vi "Sub Routing program.vi"(0 "queue Out in":refnum<queue>, 1 "FeedBack Channel":string[](array[string]), 2 "Load":refnum<vi>, 5 "reference in":refnum<vi>, 9 "Feature Step Enable":T1(array[cluster]), 11 "error in (no error)":errorcluster, 12 "Str Refnum":refnum<vi>, 13 "Lvdt":refnum<vi>, 14 "Pict Refnum":refnum<vi>) -> (3 "2D Picture":picture, 4 "Queue out":refnum<queue>, 6 "reference out":refnum<vi>, 10 "Result":bool, 15 "error out":errorcluster)   [LabVIEW 2020]
uses:
  Test  enqueue/AutoTest seq.ctl
  Galobal variable_TI.vi
  Project Setup/Globle Variable/GR_Servo.vi
panel:
  out "error out 2":errorcluster
  in  "Select Part":u16(ring) items=["CHECK BARCODE.jpg", "Difusser.jpg", "FIX BLACK PART.jpg", "FIXED PCB.jpg", "INSER KEYPAD.jpg", "IONIZE PCB.jpg", "light box ionization.jpg", "MOVE DOWN PART.jpg", "MOVING PART.jpg", "PART.jpg", "PUT PART ON FIXTURE.jpg"]
  out "Error Message":string
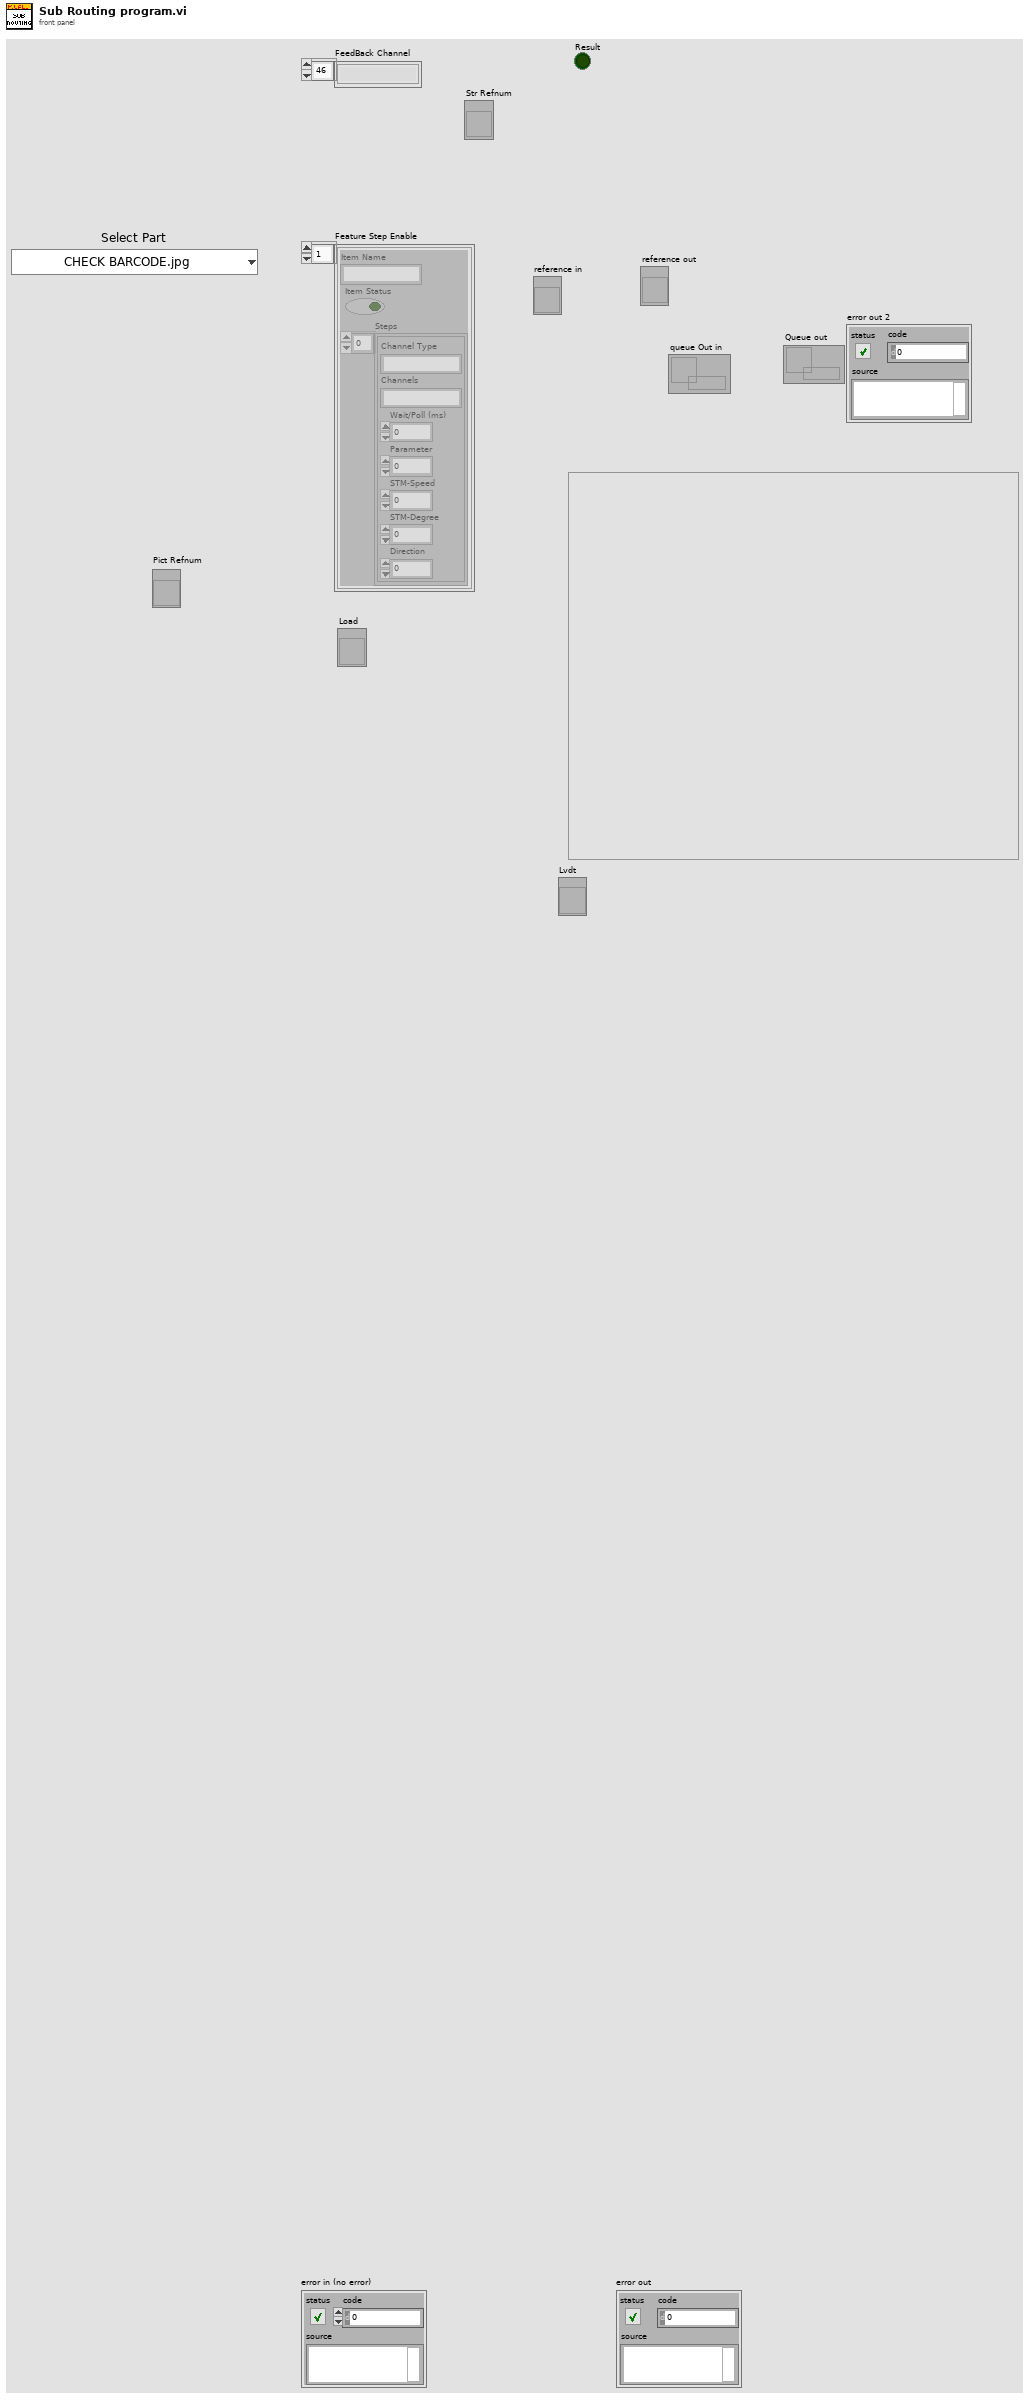
[diagram p1: front panel]
types:
  T1 = cluster{"Item Name":string, "Item Status":bool, "Steps":cluster{"Channel Type":string, "Channels":string, "Wait/Poll (ms)":u32, "Parameter":u8, "STM-Speed":i32, "STM-Degree":u32, "Direction":u8}[]}[]
  T2 = cluster{"Channel Type":string, "Channels":string, "Wait/Poll (ms)":u32, "Parameter":u8, "STM-Speed":i32, "STM-Degree":u32, "Direction":u8}[]
  T3 = cluster{"Start":bool, "Emergency ":bool, "Reset":bool, "Home":bool, "Safety":bool}
  T4 = typedef "LVPointTypeDef.ctl" = cluster{"Horizontal":i16, "Vertical":i16}
  T5 = typedef "LVBoundsTypeDef.ctl" = cluster{"Width":u32, "Height":u32}
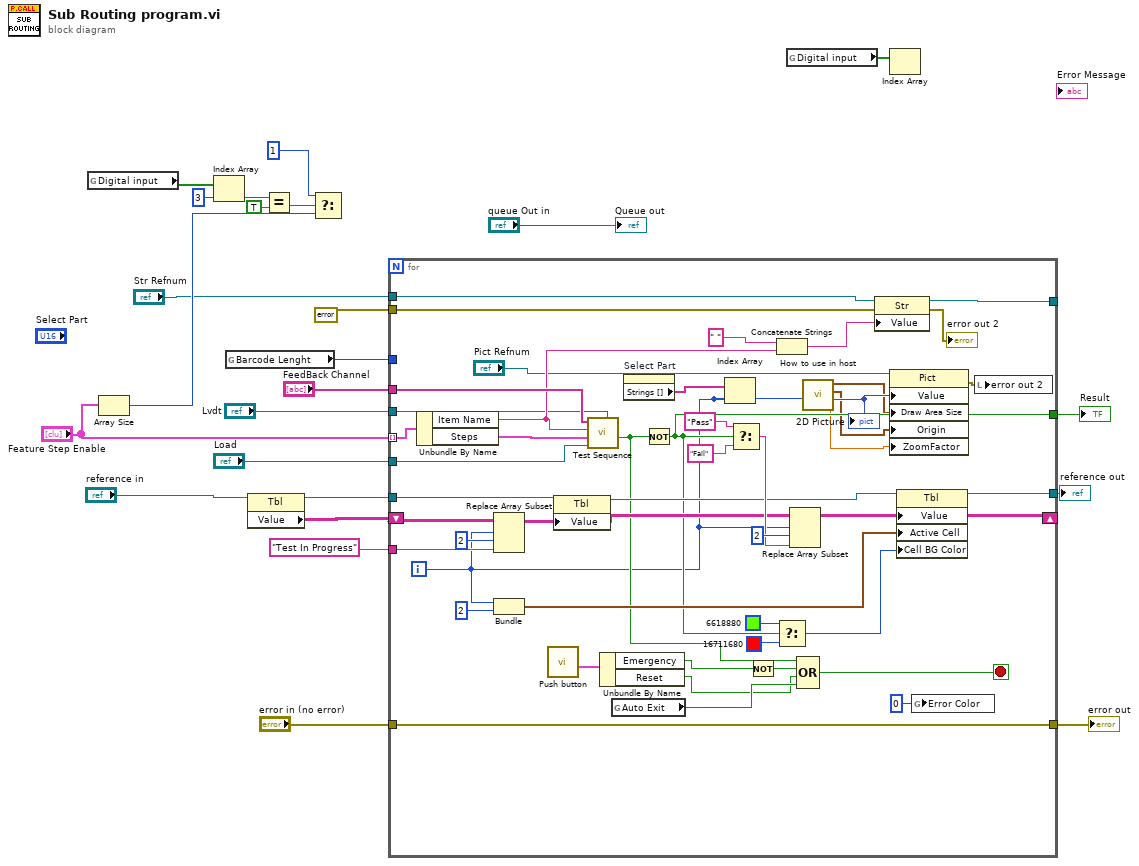
[diagram p0: block diagram]
diagram:
  n1 = global read "Galobal variable_TI.vi" "Digital input"() -> (w21:bool[])
  n2 = Array Size(array="Feature Step Enable") -> (size(s)=w6:i32)
  n3 = Index Array(array=w21, index=3) -> (element=w20:bool)
  n4 = global read "Galobal variable_TI.vi" "Barcode Lenght"() -> (w22:i32)
  n5 = property class="Tbl"(reference="reference in") -> (reference out=w10:refnum<vi>, "Value"=w13:string[][])  [unwired: 1 in, 1 out]
  n6 = Equal?(x=w20, y=TRUE) -> (x = y?=w17:bool)
  n7 = Select(t=1, s=w17, f=w6) -> ()  [unwired: 1 out]
  n8 = for {
    tunnel: "Feature Step Enable" -> [w71] mode=indexing
    tunnel: "FeedBack Channel" -> [w68]
    tunnel: w22 -> [_]
    shift-right: [w52] -> _
    shift-left: w13 -> [w64]
    tunnel: "Test In Progress" ("new element/subarray") -> [w63]
    tunnel: w10 -> [w62]
    tunnel: [w53] -> w9
    tunnel: "error in (no error)" -> [w51]
    tunnel: [w51] -> w7
    tunnel: [w46] -> w5
    tunnel: "Str Refnum" -> [w44]
    tunnel: [w43] -> _
    tunnel: errorcluster {"status"=FALSE, "code"=0, "source"=""} ("error in (no error)") -> [w37]
    tunnel: "Load" -> [w33]
    tunnel: "Lvdt" -> [w32]
    i -> [w31]
    stop <- w39 stop-if-true
    n9 = Unbundle By Name(w71) -> ("Item Name"=w41:string, "Steps"=w67:T2)
    n10 = Replace Array Subset(array=w64, new element=w63, index (row)=w31, index (col)=2 ("disabled index (col)")) -> (w59:string[][])
    n11 = Bundle(w31, 2) -> (w58:cluster{i32, i32})  [unwired: 1 in]
    n12 = call "Push button.vi"() -> ("Push Button"=w50:T3)  [unwired: 11 in]
    n13 = property class="Tbl"(reference=w62, "Value"=w59) -> (reference out=w54:refnum<vi>)  [unwired: 1 in, 1 out]
    n14 = call "Test Sequence.vi"("FeedBack Channel"=w68, "Test Name"=w41, "Steps"=w67, "Load"=w33, "Lvdt"=w32) -> ("Condition"=w47:bool)  [unwired: 2 in, 2 out]
    n15 = Unbundle By Name(w50) -> ("Emergency"=w49:bool, "Reset"=w29:bool)
    n16 = global read "Galobal variable_TI.vi" "Auto Exit"() -> (w30:bool)
    n17 = property on="Select Part" class="Ring (strict)"() -> ("Strings []"=w40:string[])  [unwired: 2 in, 2 out]
    n18 = Not(x=w47) -> (.not. x?=w46:bool)
    n19 = Index Array(array=w40, index=w31) -> ()  [unwired: 1 out]
    n20 = Select(t="Pass", s=w46, f="Fail") -> (s? t:f=w60:string)
    n21 = Not(x=w49) -> (.not. x?=w48:bool)
    n22 = Concatenate Strings(" " ("string"), w41) -> (w42:string)
    n23 = Select(t=u32 6618880 ("Color Box"), s=w46, f=u32 16711680 ("Color Box")) -> (s? t:f=w55:u32)
    n24 = Replace Array Subset(array=w59, new element=w60, index (row)=w31, index (col)=2 ("disabled index (col)")) -> (w52:string[][])
    n25 = Compound Arithmetic op=OR(w47, w48, w29, w30) -> (w39:bool)
    n26 = call "How to use in host.vi"("Select Part"=w31) -> ("zoom"=w25:sgl, "2D Picture"=w36:picture, "output cluster"=w26:T4, "Draw Area Size"=w27:T5)  [unwired: 7 in]
    "2D Picture" <- w36
    n27 = property class="Str"(reference=w44, error in=w37, "Value"=w42) -> (reference out=w43:refnum<vi>, error out=→"error out 2":errorcluster)
    n28 = property class="Pict"(reference="Pict Refnum", "Value"=w36, "Draw Area Size"=w27, "Origin"=w26, "ZoomFactor"=w25) -> (error out=w34:errorcluster)  [unwired: 1 in, 1 out]
    n29 = property class="Tbl"(reference=w54, "Value"=w52, "Active Cell"=w58, "Cell BG Color"=w55) -> (reference out=w53:refnum<vi>)  [unwired: 1 in, 1 out]
    n30 = global write "GR_Servo.vi" "Error Color"(0 ("Error Color")) -> ()
    n31 = local write "error out 2"(w34) -> ()
  }
  "error out" <- w7
  "reference out" <- w9
  "Result" <- w5
  n32 = global read "Galobal variable_TI.vi" "Digital input"() -> (w23:bool[])
  n33 = Index Array(array=w23) -> ()  [unwired: 1 in, 1 out]
  "Queue out" <- "queue Out in"
